vi "3D_ini (SubVI).vi"(8 "error in (no error)":errorcluster) -> (3 "SceneObject out":refnum<vi>)   [LabVIEW 2017]
uses:
  <vilib>/picture/3D Picture Control/Object/Create Object (name).vi
  <vilib>/picture/3D Picture Control/Object/Add Object (no reference).vi
  <vilib>/picture/3D Picture Control/Object/Create Object (drawable).vi
  <vilib>/picture/3D Picture Control/NI_3D Picture Control.lvlib
  <vilib>/picture/3D Picture Control/Helpers/Apply Texture (no reference).vi
  <vilib>/picture/3D Picture Control/Helpers/Set Clip Plane (no reference).vi
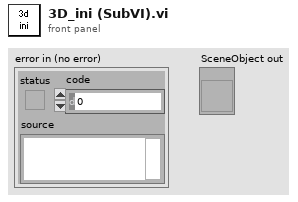
[diagram p1: front panel]
types:
  T1 = cluster{"Red":sgl, "Green":sgl, "Blue":sgl, "Alpha":sgl}
  T2 = typedef "imagedata.ctl" = cluster{"image type":i32, "image depth":i32, "image":u8[], "mask":u8[], "colors":u32[], "Rectangle":cluster{"left":i16, "top":i16, "right":i16, "bottom":i16}}
  T3 = enum16{"As a Decal", "With Modulation", "With Blending", "As a replacement"}
  T4 = cluster{"element":dbl, "element":dbl, "element":dbl}
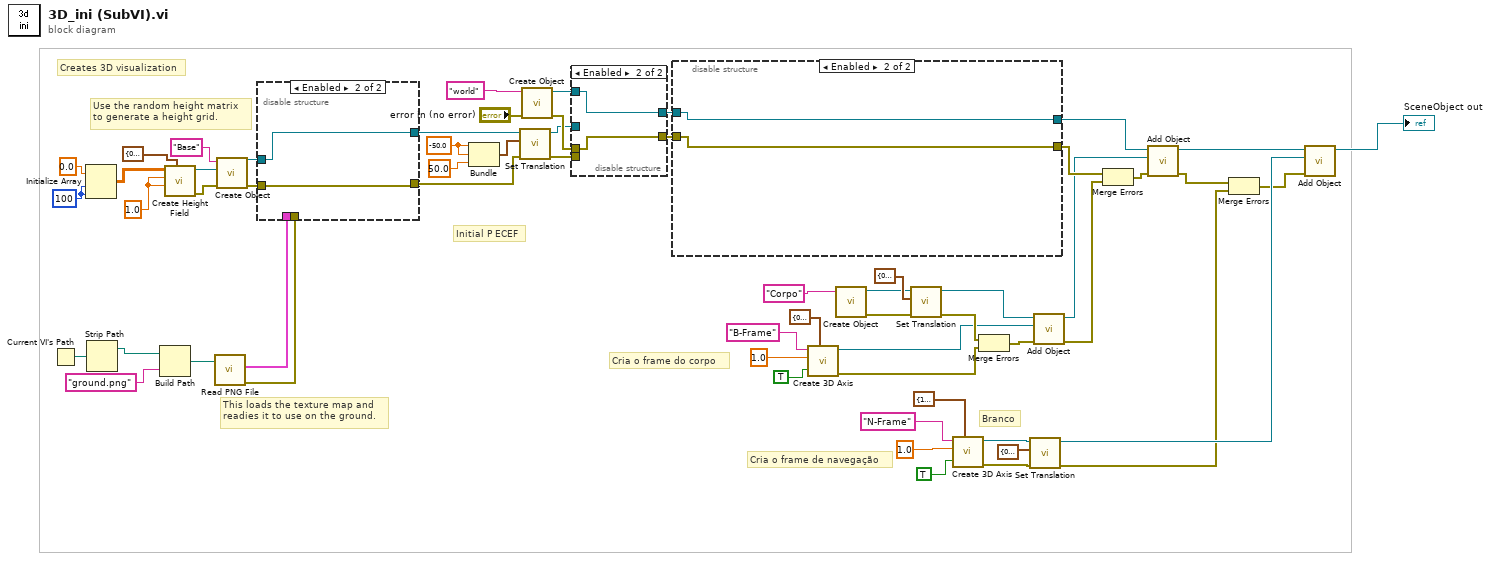
[diagram p0: block diagram]
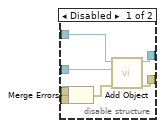
[diagram p2: hidden frame]
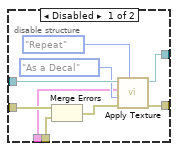
[diagram p3: hidden frame]
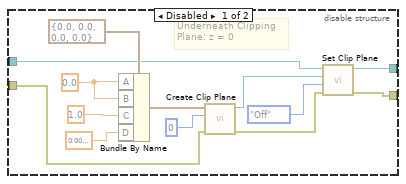
[diagram p4: hidden frame]
diagram:
  w1 = sgl 1.0 ("Length Y")
  w52 = -50.0 ("element")
  w9 = 100 ("dimension size")
  # "This loads the texture map and\nreadies it to use on the ground."
  # "Creates 3D visualization"
  # "Initial P ECEF"
  # "Branco"
  # "Cria o frame do corpo"
  # "Cria o frame de navegação"
  # "Use the random height matrix\nto generate a height grid."
  n1 = Current VI's Path() -> (path=w5:path)
  n2 = Initialize Array(sgl 0.0 ("element"), w9, w9) -> (w2:sgl[][])
  n3 = Strip Path(path=w5) -> (stripped path=w6:path)  [unwired: 1 out]
  n4 = Build Path(base path=w6, name or relative path="ground.png") -> (appended path=w7:path)
  n5 = call <vilib>:"Create Height Field.vi"("Color"=T1 {"Red"=0.0, "Green"=1.0, "Blue"=0.0, "Alpha"=1.0}, "Column Interval"=w1, "Row Interval"=w1, "Data"=w2) -> ("error out"=w58:errorcluster, "New Height Field Refnum"=w59:refnum<vi>)  [unwired: 6 in]
  n6 = call <vilib>:"Read PNG File.vi"("path to PNG file"=w7) -> ("error out"=w19:errorcluster, "image data"=w12:T2)  [unwired: 8 in, 1 out]
  n7 = call-poly <vilib>:"Create Object.vi"("error in (no error)"=w58, "Geometry"=w59, "Name"="Base") -> ("error out"=w60:errorcluster, "Scene:New Object"=w57:refnum<vi>)  [unwired: 7 in]
  n8 = disable-structure shown="Enabled" {
    disable-tunnel: w60 -> [w69 w70]
    disable-tunnel: w57 -> [w68 w71]
    disable-tunnel: w19 -> [w64 _]
    disable-tunnel: [w63 w70] -> w18
    disable-tunnel: w12 -> [w62 _]
    disable-tunnel: [w61 w71] -> w11
    frame Disabled {
      n9 = Merge Errors(w69, w64) -> (w67:errorcluster)
      n10 = call-poly <vilib>:"Apply Texture.vi"("Horizontal Wrap Mode"=enum16{"Clamp", "Repeat"}."Repeat", "error in (no error)"=w67, "Apply Mode"=T3."As a Decal", "Image Data"=w62, "Scene Object In"=w68) -> ("error out"=w63:errorcluster, "Scene Object Out"=w61:refnum<vi>)  [unwired: 5 in]
    }
    frame Enabled {
    }
  }
  n11 = Bundle("element"=w52, "element"=w52, "element"=50.0) -> (w8:T4)  [unwired: 1 out]
  n12 = call <vilib>:"Set Translation.vi"("error in (no error)"=w18, "Translation"=w8, "Scene Object"=w11) -> ("error out"=w17:errorcluster, "Translated Object"=w14:refnum<vi>)  [unwired: 7 out]
  n13 = call-poly <vilib>:"Create Object.vi"("error in (no error)"="error in (no error)", "Name"="world") -> ("error out"=w16:errorcluster, "Scene:New Object"=w15:refnum<vi>)  [unwired: 8 in]
  n14 = disable-structure shown="Enabled" {
    disable-tunnel: [w78 w79] -> w55
    disable-tunnel: [w77 w80] -> w54
    disable-tunnel: w17 -> [w75 _]
    disable-tunnel: w16 -> [w74 w79]
    disable-tunnel: w15 -> [w73 w80]
    disable-tunnel: w14 -> [w72 _]
    frame Disabled {
      n15 = Merge Errors(w74, w75) -> (w76:errorcluster)
      n16 = call-poly <vilib>:"Add Object.vi"("error in (no error)"=w76, "New Object In"=w72, "Scene Object In"=w73) -> ("error out"=w78:errorcluster, "Scene Object Out"=w77:refnum<vi>)  [unwired: 7 in]
    }
    frame Enabled {
    }
  }
  n17 = disable-structure shown="Enabled" {
    disable-tunnel: [w93 w94] -> w36
    disable-tunnel: [w92 w95] -> w37
    disable-tunnel: w54 -> [w82 w95]
    disable-tunnel: w55 -> [w81 w94]
    frame Disabled {
      w91 = sgl 0.0 ("A")
      # "Underneath Clipping\nPlane: z = 0"
      n18 = Bundle By Name(cluster=cluster{"A":sgl, "B":sgl, "C":sgl, "D":sgl} {"A"=0.0, "B"=0.0, "C"=0.0, "D"=0.0} ("Plane"), "A"=w91, "B"=w91, "C"=sgl 1.0 ("B"), "D"=sgl 0.01 ("B")) -> (w88:cluster{"A":sgl, "B":sgl, "C":sgl, "D":sgl})
      n19 = call <vilib>:"Create Clip Plane.vi"("error in (no error)"=w81, "Number"=0, "Plane"=w88) -> ("error out"=w84:errorcluster, "New Clip Plane Refnum"=w86:refnum<vi>)  [unwired: 7 out]
      n20 = call-poly <vilib>:"Set Clip Plane.vi"("error in (no error)"=w84, "Clip Plane State"=enum16{"Inherit Value", "Off", "On"}."Off", "Clip Plane Refnum In"=w86, "Scene Object In"=w82) -> ("error out"=w93:errorcluster, "Scene Object Out"=w92:refnum<vi>)  [unwired: 6 in]
    }
    frame Enabled {
    }
  }
  n21 = call <vilib>:"Create 3D Axis.vi"("Axis label?"=TRUE, "Color"=T1 {"Red"=0.0, "Green"=1.0, "Blue"=0.0, "Alpha"=1.0}, "Length"=sgl 1.0 ("Radius"), "Name"="B-Frame") -> ("error out"=w35:errorcluster, "New Object Refnum"=w34:refnum<vi>)  [unwired: 6 in]
  n22 = call-poly <vilib>:"Create Object.vi"("Name"="Corpo") -> ("error out"=w41:errorcluster, "Scene:New Object"=w40:refnum<vi>)  [unwired: 9 in]
  n23 = call <vilib>:"Set Translation.vi"("error in (no error)"=w41, "Translation"=cluster{"X":sgl, "Y":sgl, "Z":sgl} {"X"=0.0, "Y"=0.0, "Z"=0.0}, "Scene Object"=w40) -> ("error out"=w38:errorcluster, "Translated Object"=w39:refnum<vi>)  [unwired: 7 out]
  n24 = call <vilib>:"Create 3D Axis.vi"("Axis label?"=TRUE, "Color"=T1 {"Red"=1.0, "Green"=1.0, "Blue"=1.0, "Alpha"=1.0}, "Length"=sgl 1.0 ("Radius"), "Name"="N-Frame") -> ("error out"=w44:errorcluster, "New Object Refnum"=w45:refnum<vi>)  [unwired: 6 in]
  n25 = Merge Errors(w38, w35) -> (w31:errorcluster)
  n26 = call <vilib>:"Set Translation.vi"("error in (no error)"=w44, "Translation"=cluster{"X":sgl, "Y":sgl, "Z":sgl} {"X"=0.0, "Y"=0.0, "Z"=0.0}, "Scene Object"=w45) -> ("error out"=w46:errorcluster, "Translated Object"=w47:refnum<vi>)  [unwired: 7 out]
  n27 = call-poly <vilib>:"Add Object.vi"("error in (no error)"=w31, "New Object In"=w34, "Scene Object In"=w39) -> ("error out"=w33:errorcluster, "Scene Object Out"=w32:refnum<vi>)  [unwired: 7 in]
  n28 = Merge Errors(w36, w33) -> (w21:errorcluster)
  n29 = call-poly <vilib>:"Add Object.vi"("error in (no error)"=w21, "New Object In"=w32, "Scene Object In"=w37) -> ("error out"=w27:errorcluster, "Scene Object Out"=w24:refnum<vi>)  [unwired: 7 in]
  n30 = Merge Errors(w27, w46) -> (w28:errorcluster)
  n31 = call-poly <vilib>:"Add Object.vi"("error in (no error)"=w28, "New Object In"=w47, "Scene Object In"=w24) -> ("Scene Object Out"=→"SceneObject out":refnum<vi>)  [unwired: 7 in, 1 out]
